vi "Read PubDataEvents.vi"(11 "UserEvents in":refnum<class "UserEvents.lvclass">) -> (2 "PubDataEvents":T1, 3 "UserEvents out":refnum<class "UserEvents.lvclass">)   [LabVIEW 2013, in "UserEvents.lvclass"]
uses:
  UserEvents.lvclass
  Typedefs/PubDataEvents.ctl
  Typedefs/StateSelector.ctl
  <userlib>/Common/ILC/Typedefs/OutputData.ctl
  <userlib>/Common/ILC/Typedefs/InputData.ctl
  <userlib>/Common/ILC/Configuration/InputChannels.ctl
  <userlib>/Common/ILC/Typedefs/LimitSwitches.ctl
  <userlib>/Common/ILC/Typedefs/ADCs.ctl
  <userlib>/Common/ILC/Configuration/ILCConfig.ctl
  <userlib>/Common/ILC/Configuration/ScanRate_Hz_MultichannelOptions.ctl
  UserEvents.lvclass/UserEvents.ctl
  <userlib>/Common/ILC/Typedefs/ILCTypedefs.lvlib
  <userlib>/Common/ILC/Configuration/ILCConfiguration.lvlib
panel:
  # "DAC"
  # "Limit Switches"
  # "ADCs"
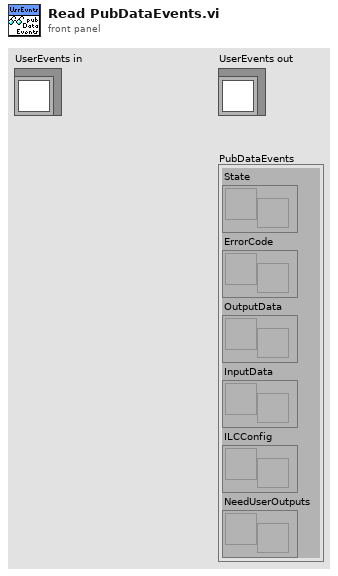
[diagram p1: front panel]
types:
  T1 = typedef "PubDataEvents.ctl" = cluster{"State":refnum<user-event>, "ErrorCode":refnum<user-event>, "OutputData":refnum<user-event>, "InputData":refnum<user-event>, "ILCConfig":refnum<user-event>, "NeedUserOutputs":refnum<user-event>}
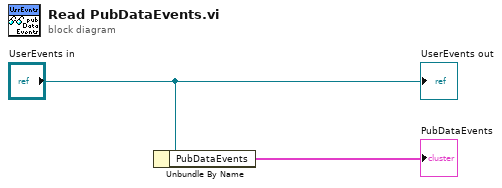
[diagram p0: block diagram]
diagram:
  n1 = Unbundle By Name("UserEvents in") -> ("PubDataEvents"=→"PubDataEvents":T1)
  "UserEvents out" <- "UserEvents in"
